vi "VIG Valid Connection IDs.vi"(7 "Method (Read)":T1, 8 "error in (no error)":errorcluster, 9 "Page":string, 10 "Tick Of Reply":u32, 11 "Connection ID":u64) -> (0 "error out":errorcluster, 1 "Pages":string[](array[string]), 2 "Ticks":u32[](array[numeric]), 3 "Connections":u64[](array[numeric]))   [LabVIEW 2015, in "Front Panel Publisher.lvlib" / "Front Panel Manager.lvclass"]
doc: "This VI is a functional global that keeps track of valid Connection IDs, the pages they requested, and the time of the last event with that page and connection."
uses:
  Front Panel Manager.lvclass
  Connection ID Methods.ctl
  <userlib>/_OpenG.lib/array/array.llb/Remove Duplicates from 1D Array (U64)__ogtk.vi
  <userlib>/_OpenG.lib/array/array.llb/Delete Elements from 1D Array (String)__ogtk.vi
  <userlib>/_OpenG.lib/array/array.llb/Delete Elements from 1D Array (U32)__ogtk.vi
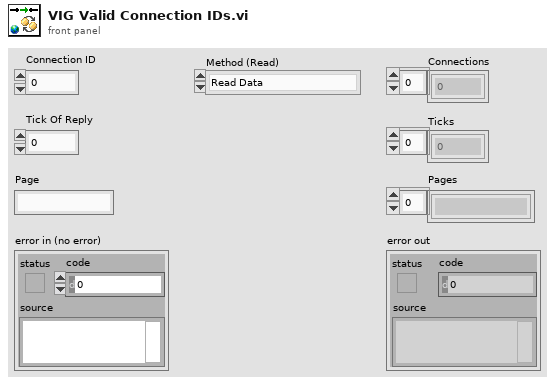
[diagram p1: front panel]
types:
  T1 = typedef "Front Panel Publisher.lvlib/Front Panel Manager.lvclass/Connection ID Methods.ctl" = enum16{"Read Data", "Write Connection ID", "Remove Connection ID"}
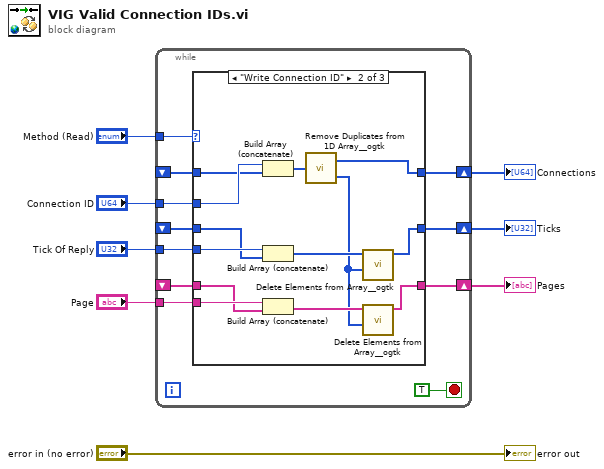
[diagram p0: block diagram]
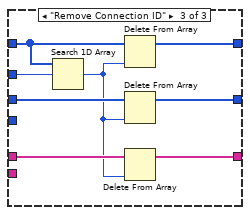
[diagram p3: hidden frame]
diagram:
  n1 = while {
    tunnel: "Method (Read)" -> [w19]
    tunnel: "Connection ID" -> [w18]
    shift-right: [w17] -> w3
    shift-left: _ -> [w16]
    tunnel: "Tick Of Reply" -> [w14]
    shift-right: [w13] -> w4
    shift-left: _ -> [w12]
    tunnel: "Page" -> [w11]
    shift-right: [w10] -> w1
    shift-left: _ -> [w9]
    stop <- TRUE stop-if-true
    n2 = case shown="\"Write Connection ID\"" w19 {
      tunnel: w18 -> [_ w35 w43]
      tunnel: [w22 w33 w39] -> w17
      tunnel: w16 -> [w22 w34 w40]
      tunnel: w14 -> [_ w31 _]
      tunnel: [w21 w28 w41] -> w13
      tunnel: w12 -> [w21 w30 w42]
      tunnel: w11 -> [_ w27 _]
      tunnel: [w20 w24 w36] -> w10
      tunnel: w9 -> [w20 w26 w38]
      frame "Read Data" {
      }
      frame "Write Connection ID" {
        n3 = Build Array (concatenate)(w35, w34) -> (w32:u64[])
        n4 = Build Array (concatenate)(w31, w30) -> (w29:u32[])
        n5 = Build Array (concatenate)(w27, w26) -> (w25:string[])
        n6 = call-poly <userlib>:"Remove Duplicates from 1D Array__ogtk.vi"("Input Array"=w32) -> ("Output Array"=w33:u64[], "indices of removed elements"=w23:i32[])
        n7 = call-poly <userlib>:"Delete Elements from Array__ogtk.vi"("indices"=w23, "array"=w29) -> ("array w/ subset deleted"=w28:u32[])  [unwired: 8 in, 1 out]
        n8 = call-poly <userlib>:"Delete Elements from Array__ogtk.vi"("indices"=w23, "array"=w25) -> ("array w/ subset deleted"=w24:string[])  [unwired: 8 in, 1 out]
      }
      frame "Remove Connection ID" {
        n9 = Search 1D Array(1D array=w40, element=w43) -> (index of element=w37:i32)  [unwired: 1 in]
        n10 = Delete From Array(array=w40, index=w37) -> (array with subset deleted=w39:u64[])  [unwired: 1 in, 1 out]
        n11 = Delete From Array(array=w42, index=w37) -> (array with subset deleted=w41:u32[])  [unwired: 1 in, 1 out]
        n12 = Delete From Array(array=w38, index=w37) -> (array with subset deleted=w36:string[])  [unwired: 1 in, 1 out]
      }
    }
  }
  "Ticks" <- w4
  "Connections" <- w3
  "Pages" <- w1
  "error out" <- "error in (no error)"
